vi "Fetch.vi"(8 "error in (no error)":errorcluster, 10 "Message in":refnum<class "FetchMessage.lvclass">, 11 "ExampleClassC in":refnum<class "ExampleClassC.lvclass">) -> (0 "error out":errorcluster, 3 "ExampleClassC out":refnum<class "ExampleClassC.lvclass">)   [LabVIEW 2012, in "ExampleClassC.lvclass"]
doc: "The fetch method processes the command 'fetch'.\n\nThe command 'fetch' is used for receiving various forms of data."
uses:
  ExampleClassC.lvclass
  <vilib>/Distrio/Murmex/FetchMessage/FetchMessage.lvclass
  <vilib>/Distrio/Murmex/Murmex/Murmex.lvclass
  <vilib>/Distrio/Murmex/Message/Message.lvclass
panel:
  # "This method is called when the FETCH\ntrigger is sent. \n\nOverride this method when your component needs to\nrespond to this trigger. \n\nCall parent for proper implementation"
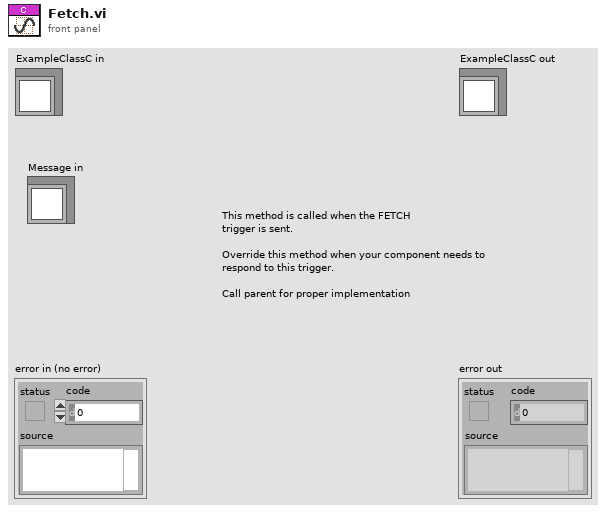
[diagram p1: front panel]
types:
  T1 = typedef "Image Type" = u32
  T2 = typedef "Murmex.lvlib/Murmex.lvclass/observer_cluster_2.ctl" = cluster{"ID":string, "observe mode":T3, "channels":string, "queue type":T4, "wait until done?":bool}
  T3 = typedef "Murmex.lvlib/Murmex.lvclass/observe_mode_enum.ctl" = enum16{"all data blocks", "only finished data blocks"}
  T4 = typedef "Murmex.lvlib/Murmex.lvclass/Queue type enum.ctl" = enum16{"RabbitMQ", "Network streaming queue"}
  T5 = typedef "Murmex.lvlib/FetchMessage.lvclass/Channel data cluster.ctl" = cluster{"channel id":i32, "data UInt8":u8[], "data type":T6, "dimensions":i32[], "physical units":T7[], "waveform dt":dbl, "waveform":T8}
  T6 = typedef "Murmex.lvlib/Murmex.lvclass/data_type_enum.ctl" = enum16{"Float128", "Float64", "Float32", "Int64", "Int32", "Int16", "Int8", "UInt64", "UInt32", "UInt16", "UInt8", "Boolean", "String"}
  T7 = typedef "Murmex.lvlib/Murmex.lvclass/Physical Units.ctl" = cluster{"Base Units":enum16{"radian", "steradian", "second", "meter", "kilogram", "ampere", "kelvin", "mole", "candela"}, "Exponent":i16}
  T8 = typedef "Murmex.lvlib/Murmex.lvclass/waveform_type_enum.ctl" = enum16{"no waveform", "analog", "digital"}
  T9 = typedef "IMAQ Image.ctl" = refnum<image>
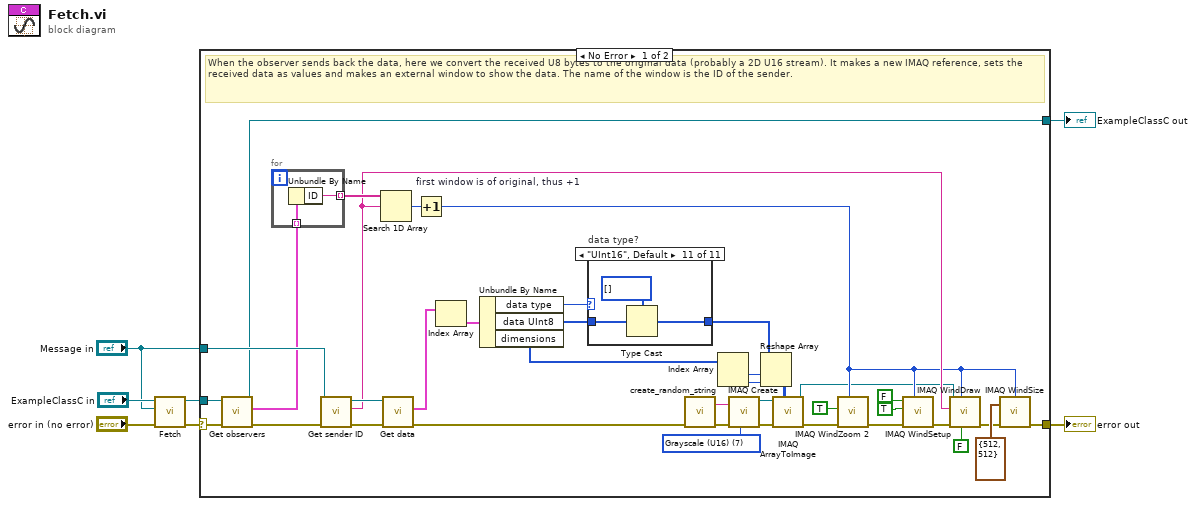
[diagram p0: block diagram]
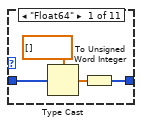
[diagram p2: hidden frame]
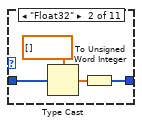
[diagram p3: hidden frame]
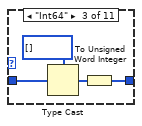
[diagram p4: hidden frame]
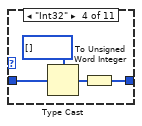
[diagram p5: hidden frame]
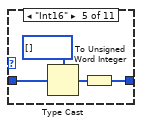
[diagram p6: hidden frame]
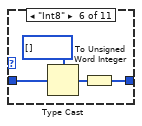
[diagram p7: hidden frame]
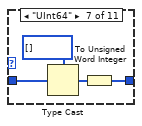
[diagram p8: hidden frame]
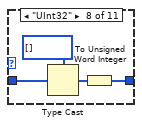
[diagram p9: hidden frame]
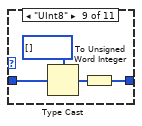
[diagram p10: hidden frame]
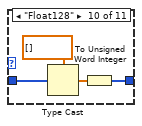
[diagram p11: hidden frame]
diagram:
  n1 = call-parent "Fetch.vi"("error in (no error)"="error in (no error)", "Message in"="Message in", "Murmex in"="ExampleClassC in") -> ("error out"=w5:errorcluster, "Murmex out"=w1:refnum<class "ExampleClassC.lvclass">)  [unwired: 7 in]
  n2 = case shown="No Error" w5 {
    selector: w5 -> [w43 w92]
    tunnel: "Message in" -> [w40 _]
    tunnel: [w42 w92] -> w4
    tunnel: w1 -> [w37 w91]
    tunnel: [w36 w91] -> w3
    frame No Error {
      w21 = T1 7 items=["Grayscale (U8)", "Grayscale (I16)", "Grayscale (SGL)", "Complex (CSG)", "RGB (U32)", "HSL (U32)", "RGB (U64)", "Grayscale (U16)"] ("Image Type")
      # "When the observer sends back the data, here we convert the received U8 bytes to the original data (probably a 2D U16 stream). It makes a new IMAQ reference, sets the received data as values and makes an external window to show the data. The name of the window is the ID of the sender."
      n3 = call <vilib>:"Get observers.vi"("error in (no error)"=w43, "Murmex in"=w37) -> ("error out"=w38:errorcluster, "observers (component IDs)"=w35:T2[], "Murmex out"=w36:refnum<class "ExampleClassC.lvclass">)  [unwired: 7 in]
      n4 = for {
        tunnel: w35 -> [w90] mode=indexing
        tunnel: [w89] -> w34 mode=indexing
        n5 = Unbundle By Name(w90) -> ("ID"=w89:string)
      }
      n6 = call <vilib>:"Get sender ID.vi"("error in (no error)"=w38, "Message in"=w40) -> ("error out"=w41:errorcluster, "sender"=w33:string, "Message out"=w39:refnum<class "FetchMessage.lvclass">)  [unwired: 7 in]
      n7 = Search 1D Array(1D array=w34, element=w33) -> (index of element=w32:i32)  [unwired: 1 in]
      n8 = call <vilib>:"Get data.vi"("error in (no error)"=w41, "FetchMessage.lvclass"=w39) -> ("error out"=w44:errorcluster, "data (channels)"=w45:T5[])  [unwired: 7 in, 1 out]
      n9 = Increment "first window is of original, thus +1"(x=w32) -> (x+1=w31:i32)
      n10 = Index Array(array=w45) -> (element=w30:T5)  [unwired: 1 in]
      n11 = Unbundle By Name(w30) -> ("data type"=w29:T6, "data UInt8"=w28:u8[], "dimensions"=w27:i32[])
      n12 = case "data type?" shown="\"UInt16\", Default" w29 {
        tunnel: w28 -> [w49 w53 w57 w61 w65 w69 w73 w77 w81 w85 w88]
        tunnel: [w46 w50 w54 w58 w62 w66 w70 w74 w78 w82 w86] -> w26
        frame "Float64" {
          n13 = Type Cast(type=dbl[] [] ("data UInt8"), x=w49) -> (*(type *) &x=w47:dbl[])
          n14 = To Unsigned Word Integer(number=w47) -> (unsigned 16bit integer=w46:u16[])
        }
        frame "Float32" {
          n15 = Type Cast(type=sgl[] [] ("data UInt8"), x=w53) -> (*(type *) &x=w51:sgl[])
          n16 = To Unsigned Word Integer(number=w51) -> (unsigned 16bit integer=w50:u16[])
        }
        frame "Int64" {
          n17 = Type Cast(type=i64[] [] ("data UInt8"), x=w57) -> (*(type *) &x=w55:i64[])
          n18 = To Unsigned Word Integer(number=w55) -> (unsigned 16bit integer=w54:u16[])
        }
        frame "Int32" {
          n19 = Type Cast(type=i32[] [] ("data UInt8"), x=w61) -> (*(type *) &x=w59:i32[])
          n20 = To Unsigned Word Integer(number=w59) -> (unsigned 16bit integer=w58:u16[])
        }
        frame "Int16" {
          n21 = Type Cast(type=i16[] [] ("data UInt8"), x=w65) -> (*(type *) &x=w63:i16[])
          n22 = To Unsigned Word Integer(number=w63) -> (unsigned 16bit integer=w62:u16[])
        }
        frame "Int8" {
          n23 = Type Cast(type=i8[] [] ("data UInt8"), x=w69) -> (*(type *) &x=w67:i8[])
          n24 = To Unsigned Word Integer(number=w67) -> (unsigned 16bit integer=w66:u16[])
        }
        frame "UInt64" {
          n25 = Type Cast(type=u64[] [] ("data UInt8"), x=w73) -> (*(type *) &x=w71:u64[])
          n26 = To Unsigned Word Integer(number=w71) -> (unsigned 16bit integer=w70:u16[])
        }
        frame "UInt32" {
          n27 = Type Cast(type=u32[] [] ("data UInt8"), x=w77) -> (*(type *) &x=w75:u32[])
          n28 = To Unsigned Word Integer(number=w75) -> (unsigned 16bit integer=w74:u16[])
        }
        frame "UInt8" {
          n29 = Type Cast(type=u8[] [] ("data UInt8"), x=w81) -> (*(type *) &x=w79:u8[])
          n30 = To Unsigned Word Integer(number=w79) -> (unsigned 16bit integer=w78:u16[])
        }
        frame "Float128" {
          n31 = Type Cast(type=ext[] [] ("data UInt8"), x=w85) -> (*(type *) &x=w83:ext[])
          n32 = To Unsigned Word Integer(number=w83) -> (unsigned 16bit integer=w82:u16[])
        }
        frame "UInt16", Default {
          n33 = Type Cast(type=u16[] [] ("data UInt8"), x=w88) -> (*(type *) &x=w86:u16[])
        }
      }
      n34 = call <vilib>:"create_random_string.vi"("error in (no error)"=w44) -> ("error out"=w22:errorcluster, "random string"=w23:string)  [unwired: 9 in]
      n35 = Index Array(array=w27) -> (element #1=w25:i32, element #2=w24:i32)  [unwired: 2 in]
      n36 = call "IMAQ Create"("Image Name"=w23, "Image Type"=w21, "error in (no error)"=w22) -> ("New Image"=w20:T9, "error out"=w19:errorcluster)  [unwired: 2 in]
      n37 = Reshape Array(w26, w25, w24) -> (w18:u16[][])
      n38 = call "IMAQ ArrayToImage"("Image Pixels (U16)"=w18, "error in (no error)"=w19, "Image"=w20) -> ("error out"=w12:errorcluster, "Image Out"=w11:T9)  [unwired: 7 in]
      n39 = call "IMAQ WindZoom 2"("Window Number (0...15)"=w31, "error in (no error)"=w12, "Zoom to Fit? (False)"=TRUE) -> ("error out"=w16:errorcluster)  [unwired: 5 in, 3 out]
      n40 = call "IMAQ WindSetup"("Window Number (0...15)"=w31, "error in (no error)"=w16, "Window can close? (Yes)"=TRUE, "Window can grow? (Yes)"=FALSE) -> ("error out"=w17:errorcluster)  [unwired: 7 in]
      n41 = call "IMAQ WindDraw"("Resize to Image Size? (Y)"=FALSE, "Window Number (0...15)"=w31, "error in (no error)"=w17, "Title"=w33, "Image"=w11) -> ("error out"=w8:errorcluster)  [unwired: 5 in, 1 out]
      n42 = call "IMAQ WindSize"("error in (no error)"=w8, "Width & Height"=cluster{"Width":i32, "Height":i32} {"Width"=512, "Height"=512}, "Window Number"=w31) -> ("error out"=w42:errorcluster)  [unwired: 3 in, 2 out]
    }
    frame Error {
    }
  }
  "error out" <- w4
  "ExampleClassC out" <- w3
